vi "SS2 Live_Sensor Size.vi"() -> (1 "Y size":i32=256, 3 "X size":i32=512)   [LabVIEW 2019]
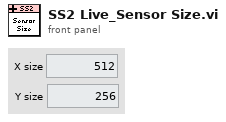
[diagram p1: front panel]
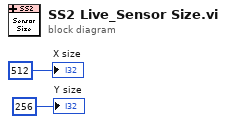
[diagram p0: block diagram]
diagram:
  "X size" <- 512 ("X size")
  "Y size" <- 256 ("Y size")
